vi "Modify_Cost_F()_Making_Different-1.vi"(1 "[IN] Cost functions":i8[](array[numeric])) -> (0 "[OUT] Cost functions":i8[](array[numeric]))   [LabVIEW 2013]
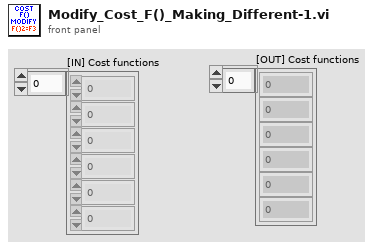
[diagram p1: front panel]
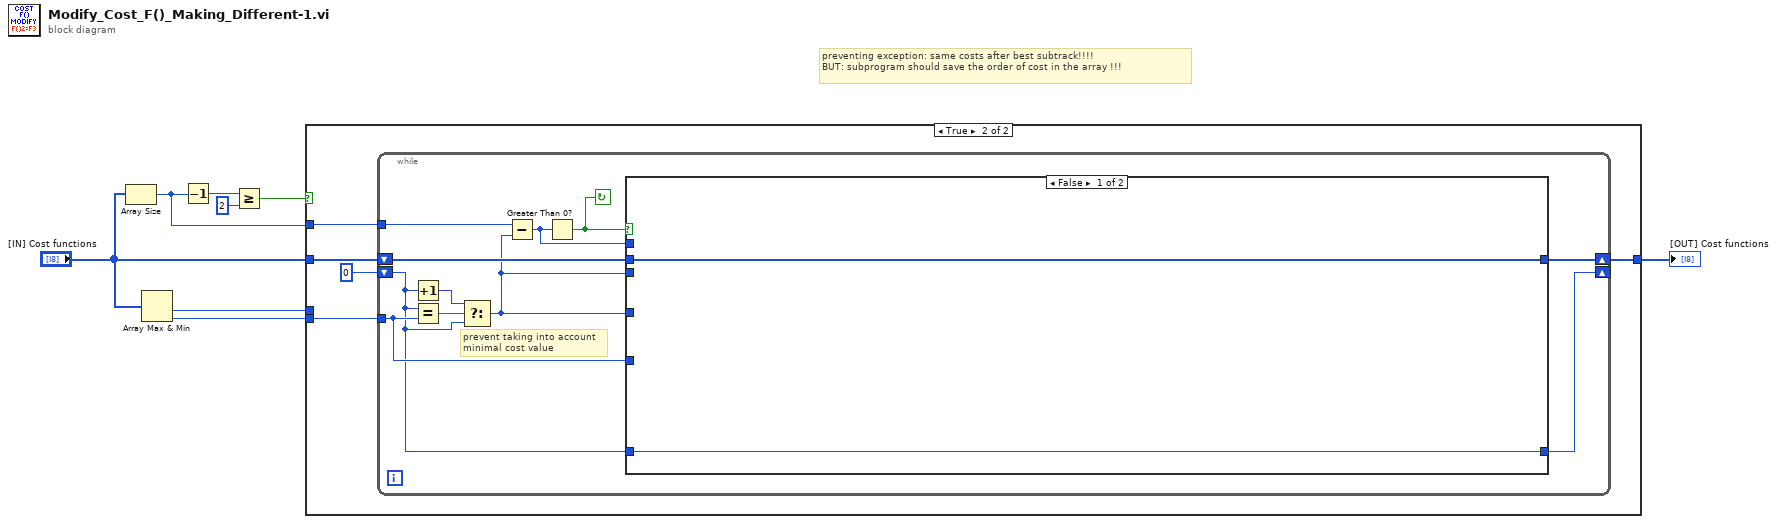
[diagram p0: block diagram]
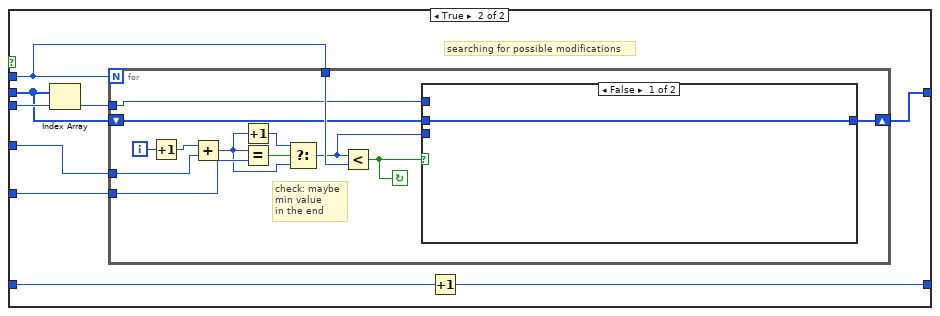
[diagram p3: hidden frame]
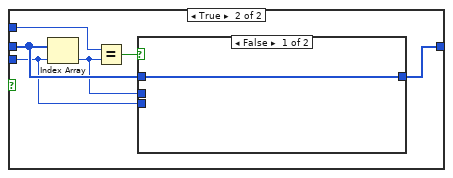
[diagram p4: hidden frame]
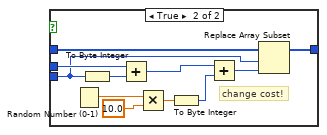
[diagram p5: hidden frame]
diagram:
  # "preventing exception: same costs after best subtrack!!!!\nBUT: subprogram should save the order of cost in the array !!!"
  n1 = Array Size(array="[IN] Cost functions") -> (size(s)=w5:i32)
  n2 = Array Max & Min(array="[IN] Cost functions") -> (min value=w1:i8, min index (indices)=w2:i32)  [unwired: 2 out]
  n3 = Decrement(x=w5) -> (x-1=w8:i32)
  n4 = Greater Or Equal?(x=w8, y=2) -> (x >= y?=w6:bool)
  n5 = case shown="True" w6 {
    tunnel: "[IN] Cost functions" -> [w9 w14]
    tunnel: w5 -> [_ w12]
    tunnel: [w9 w11] -> w4
    tunnel: w2 -> [_ w10]
    tunnel: w1 -> [_ _]
    frame False {
    }
    frame True {
      n6 = while {
        shift-right: [w17] -> w11
        shift-left: w14 -> [w21]
        shift-right: [w15] -> _
        shift-left: 0 -> [w16]
        tunnel: w12 -> [w23]
        tunnel: w10 -> [w18]
        stop <- w22 continue-if-true
        # "prevent taking into account\nminimal cost value"
        n7 = Increment(x=w16) -> (x+1=w24:i32)
        n8 = Equal?(x=w16, y=w18) -> (x = y?=w25:bool)
        n9 = Select(t=w24, s=w25, f=w16) -> (s? t:f=w19:i32)
        n10 = Subtract(x=w23, y=w19) -> (x-y=w20:i32)
        n11 = Greater Than 0?(x=w20) -> (x > 0?=w22:bool)
        n12 = case shown="False" w22 {
          tunnel: w21 -> [w27 w34]
          tunnel: w19 -> [_ w36]
          tunnel: w20 -> [_ w31]
          tunnel: w19 -> [_ w33]
          tunnel: w18 -> [_ w32]
          tunnel: [w27 w30] -> w17
          tunnel: w16 -> [w26 w29]
          tunnel: [w26 w28] -> w15
          frame False {
          }
          frame True {
            # "searching for possible modifications"
            n13 = Index Array(array=w34, index=w36) -> (element=w35:i8)
            n14 = for {
              N: w31 -> [_]
              tunnel: w35 -> [w38]
              shift-right: [w37] -> w30
              shift-left: w34 -> [w40]
              tunnel: w33 -> [w47]
              tunnel: w32 -> [w46]
              tunnel: w31 -> [w42]
              i -> [w49]
              stop <- w41 continue-if-true
              # "check: maybe \nmin value\nin the end"
              n15 = Increment(x=w49) -> (x+1=w48:i32)
              n16 = Add(x=w48, y=w47) -> (x+y=w43:i32)
              n17 = Increment(x=w43) -> (x+1=w44:i32)
              n18 = Equal?(x=w43, y=w46) -> (x = y?=w45:bool)
              n19 = Select(t=w44, s=w45, f=w43) -> (s? t:f=w39:i32)
              n20 = Less?(x=w39, y=w42) -> (x < y?=w41:bool)
              n21 = case shown="False" w41 {
                tunnel: w40 -> [w50 w54]
                tunnel: w39 -> [_ w53]
                tunnel: w38 -> [_ w56]
                tunnel: [w50 w51] -> w37
                frame False {
                }
                frame True {
                  n22 = Index Array(array=w54, index=w53) -> (element=w52:i8)
                  n23 = Equal?(x=w56, y=w52) -> (x = y?=w55:bool)
                  n24 = case shown="False" w55 {
                    tunnel: w54 -> [w57 w61]
                    tunnel: w53 -> [_ w59]
                    tunnel: w52 -> [_ w62]
                    tunnel: [w57 w58] -> w51
                    frame False {
                    }
                    frame True {
                      # "change cost!"
                      n25 = Random Number (0-1)() -> (number: 0 to 1=w67:dbl)
                      n26 = To Byte Integer(number=w59) -> (8bit integer=w68:i8)
                      n27 = Add(x=w62, y=w68) -> (x+y=w64:i8)
                      n28 = Multiply(x=w67, y=10.0) -> (x*y=w65:dbl)
                      n29 = To Byte Integer(number=w65) -> (8bit integer=w63:i8)
                      n30 = Add(x=w64, y=w63) -> (x+y=w60:i8)
                      n31 = Replace Array Subset(array=w61, new element=w60, index=w59) -> (w58:i8[])
                    }
                  }
                }
              }
            }
            n32 = Increment(x=w29) -> (x+1=w28:i32)
          }
        }
      }
    }
  }
  "[OUT] Cost functions" <- w4
